vi "Main.vi"() -> ()   [LabVIEW 2022 SP3]
uses:
  States/FSM States V2.ctl
  <vilib>/express/express arith-compare/Formula/XNode/ExpressFormulaBlockNode.xnode
panel:
  out "Flag data log":i32=1 min=1 max=10 step=1
  out "Pitch positions (deg)":T1(graph)
  out "Yaw positions (deg)":T2(graph)
  in  "Start":bool
  in  "Load Button":bool
  in  "Default Button":bool
  out "Current state":T3
  in  "Stop button":bool
  in  "Tab Control":T4(tab)
  in  "Init Controller Parameters":T5={"Resolution level, N"=1, "Samples, re"=1, "Yaw gains"=[], "Pitch rate, mK"=[], "Yaw rate, mK"=[], "Pitch gains"=[], "Type controller, TC"=enum."PID"} {"Pitch gains" format="%.3f"; "Yaw rate, mK" format="%.2e"; "Pitch rate, mK" format="%.2e"; "Yaw gains" format="%.3f"; "Samples, re" min=1 max=100 step=1; "Resolution level, N" min=1 max=10 step=1}
  in  "Init Model Parameters":cluster{"States":dbl[]} {"States" format="%.3f"}
  in  "Init Wavenet-IIR Parameters":T6={"Activation function, fn"=0, "Neurons, J"=1, "Feedbacks, Q"=1, "Feedforwards, R"=1, "Inputs, I"=1, "Outputs, P"=1, "Weights, hW"=0.0, "Feedbacks, ha"=0.0, "Forwards, hb"=0.0, "Scalings, hA"=0.0, "Shiftings, hB"=0.0, "Persistan signal, ps"=0.0} {"Persistan signal, ps" format="%.2e"; "Shiftings, hB" format="%.2e"; "Scalings, hA" format="%.2e"; "Forwards, hb" format="%.2e"; "Feedbacks, ha" format="%.2e"; "Weights, hW" format="%.2e"; "Outputs, P" min=1 max=10 step=1; "Inputs, I" min=1 max=10 step=1; "Feedforwards, R" min=1 max=10 step=1; "Feedbacks, Q" min=1 max=10 step=1; "Neurons, J" min=1 max=99 step=1; "Activation function, fn" items=["Morlet", "RASP1", "RASP2", "RASP3", "POLYWOG1", "POLYWOG2", "POLYWOG3", "POLYWOG4", "POLYWOG5", "Shannon", "Atomic", "Flat top 1", "Flat top 2", "Flat top 3", "Flat top 4", "Flat top 5", "Flat top 6", "Hanning", "Hamming", "Blackman", "Blackman-Harris"]}
  out "Comparision, Errors":T7 {"costfnc" format="%_2f"; "Derry" format="%_2f"; "Derrp" format="%_2f"; "Dpy" format="%_2f"; "Dpe" format="%_2f"; "Cost func" scale=1.0..1000.0; "Yaw, err" scale=-3.0..3.0; "Pitch, err" scale=-3.0..3.0; "Yaw, e" scale=-3.0..3.0; "Pitch, e" scale=-3.0..3.0}
  out "Operation Parameters":T8={"Control signal, Vq"=0.0, "Control signal, Vf"=0.0, "Total control, U"=1.0, "Iteration, k"=1, "Period, T"=1.0, "Instant, kT"=1.0, "control Vpp"=0.0, "control Vpy"=0.0} {"control Vpy" format="%_2f"; "control Vpp" format="%_2f"; "Instant, kT" min=1.0 max=10.0 step=1.0 format="%.3f"; "Period, T" min=1.0 max=10.0 step=1.0 format="%.3f"; "Iteration, k" min=1 max=10 step=1; "Total control, U" min=1.0 max=10.0 step=1.0 format="%.3f"; "Control signal, Vf" scale=-30.0..30.0; "Control signal, Vq" scale=-30.0..30.0}
  in  "Desired Positions, yd":cluster{"Pitch, q":dbl, "Yaw, f":dbl}={"Pitch, q"=1.0, "Yaw, f"=1.0} {"Yaw, f" min=-40.0 max=40.0 step=5.0 format="%.2f"; "Pitch, q" min=-40.0 max=40.0 step=5.0 format="%.2f"}
  out "Acquisition, y":cluster{"Pitch, q":dbl, "Yaw, f":dbl}={"Pitch, q"=1.0, "Yaw, f"=1.0} {"Yaw, f" min=-40.0 max=40.0 step=5.0 format="%.2f"; "Pitch, q" min=-40.0 max=40.0 step=5.0 format="%.2f"}
  out "Approximation, ya":cluster{"Pitch, q":dbl, "Yaw, f":dbl}={"Pitch, q"=1.0, "Yaw, f"=1.0} {"Yaw, f" min=-40.0 max=40.0 step=5.0 format="%.2f"; "Pitch, q" min=-40.0 max=40.0 step=5.0 format="%.2f"}
  out "Model Parameters":cluster{"States (rad)":dbl[]} {"States (rad)" format="%.3f"}
  out "Controller Parameters":T5={"Resolution level, N"=1, "Samples, re"=1, "Yaw gains"=[], "Pitch rate, mK"=[], "Yaw rate, mK"=[], "Pitch gains"=[], "Type controller, TC"=enum."PID"} {"Pitch gains" format="%.3f"; "Yaw rate, mK" format="%.2e"; "Pitch rate, mK" format="%.2e"; "Yaw gains" format="%.3f"; "Samples, re" min=1 max=100 step=1; "Resolution level, N" min=1 max=10 step=1}
  in  "Wavenet-IIR Outputs":T9 {"Rho, R" format="%.3f"; "Gamma, G" format="%.3f"; "Estimated, y" format="%.3f"; "Neural, z" format="%.3f"}
  out "Wavenet-IIR Values":T10 {"Function, dy" format="%.3f"; "Function, y" format="%.3f"; "Tau, t" format="%.3f"; "Forwards, D" format="%.3f"; "Feedbacks, C" format="%.3f"; "Weights, W" format="%.3f"; "Shifts, B" format="%.3f"; "Scales, A" format="%.3f"}
  out "Wavenet-IIR Gradients":T11 {"Forwards, D" format="%.3f"; "Feedbacks, C" format="%.3f"; "Weights, W" format="%.3f"; "Shifts, B" format="%.3f"; "Scales, A" format="%.3f"}
  out "Wavenet-IIR Memories":T12 {"Activation functions, dF" format="%.3f"; "Wavenet, Z" format="%.3f"; "Tracking errors, e" format="%.3f"; "Activation functions, F" format="%.3f"; "Wavenet-IIR, Y" format="%.3f"}
  # "These values were propused by the designer."
  # "Value in radians and degrees."
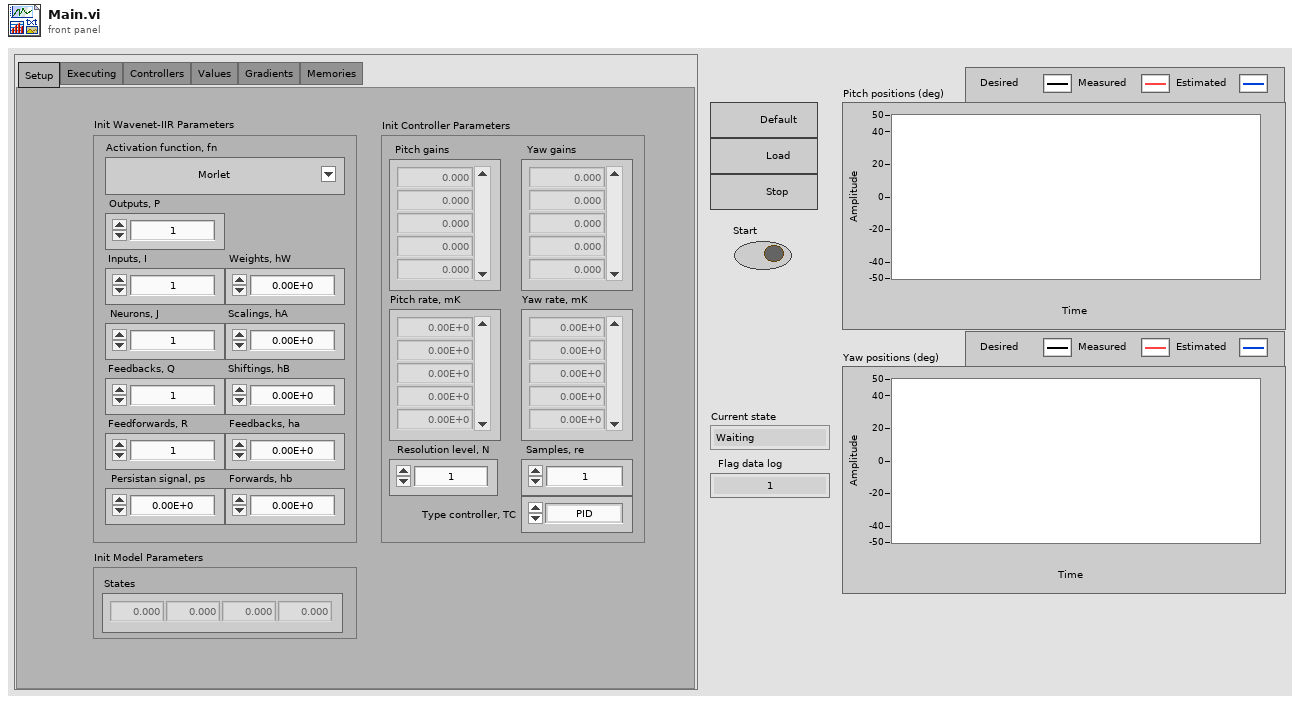
[diagram p1: front panel]
types:
  T1 = cluster{"Pitch, q":dbl, "Pitch, q":dbl, "Pitch, q":dbl}
  T2 = cluster{"Yaw, f":dbl, "Yaw, f":dbl, "Yaw, f":dbl}
  T3 = typedef "FSM States V2.ctl" = enum16{"Waiting", "Default configuration", "New configuration", "Boot parameters", "Execute", "Acquisition", "Wavelets", "WaveNet", "Filtering", "Comparision", "Gradients", "Datalog", "Update parameters", "Renew PID gains", "Renew PMR gains", "New PID signal", "New PMR signal", "Instant", "Time check", "Finish"}
  T4 = enum32{"Setup", "Executing", "Controllers", "Values", "Gradients", "Memories"}
  T5 = cluster{"Resolution level, N":i32, "Samples, re":i32, "Yaw gains":dbl[], "Pitch rate, mK":dbl[], "Yaw rate, mK":dbl[], "Pitch gains":dbl[], "Type controller, TC":enum16{"PID", "PMR"}}
  T6 = cluster{"Activation function, fn":u16, "Neurons, J":i32, "Feedbacks, Q":i32, "Feedforwards, R":i32, "Inputs, I":i32, "Outputs, P":i32, "Weights, hW":dbl, "Feedbacks, ha":dbl, "Forwards, hb":dbl, "Scalings, hA":dbl, "Shiftings, hB":dbl, "Persistan signal, ps":dbl}
  T7 = cluster{"Pitch, e":dbl, "Yaw, e":dbl, "Pitch, err":dbl, "Yaw, err":dbl, "Cost func":dbl, "Dpe":dbl, "Dpy":dbl, "Derrp":dbl, "Derry":dbl, "costfnc":dbl}
  T8 = cluster{"Control signal, Vq":dbl, "Control signal, Vf":dbl, "Total control, U":dbl, "Iteration, k":i32, "Period, T":dbl, "Instant, kT":dbl, "control Vpp":dbl, "control Vpy":dbl}
  T9 = cluster{"Neural, z":dbl[], "Estimated, y":dbl[], "Gamma, G":dbl[], "Rho, R":dbl[]}
  T10 = cluster{"Scales, A":dbl[], "Shifts, B":dbl[], "Weights, W":dbl[][], "Feedbacks, C":dbl[][], "Forwards, D":dbl[][], "Tau, t":dbl[], "Function, y":dbl[], "Function, dy":dbl[]}
  T11 = cluster{"Scales, A":dbl[], "Shifts, B":dbl[], "Weights, W":dbl[][], "Feedbacks, C":dbl[][], "Forwards, D":dbl[][]}
  T12 = cluster{"Wavenet-IIR, Y":dbl[][], "Activation functions, F":dbl[][], "Tracking errors, e":dbl[][], "Wavenet, Z":dbl[][], "Activation functions, dF":dbl[][]}
  T13 = cluster{"Pitch, q":dbl, "Pitch, q":dbl, "Numeric":dbl}[]
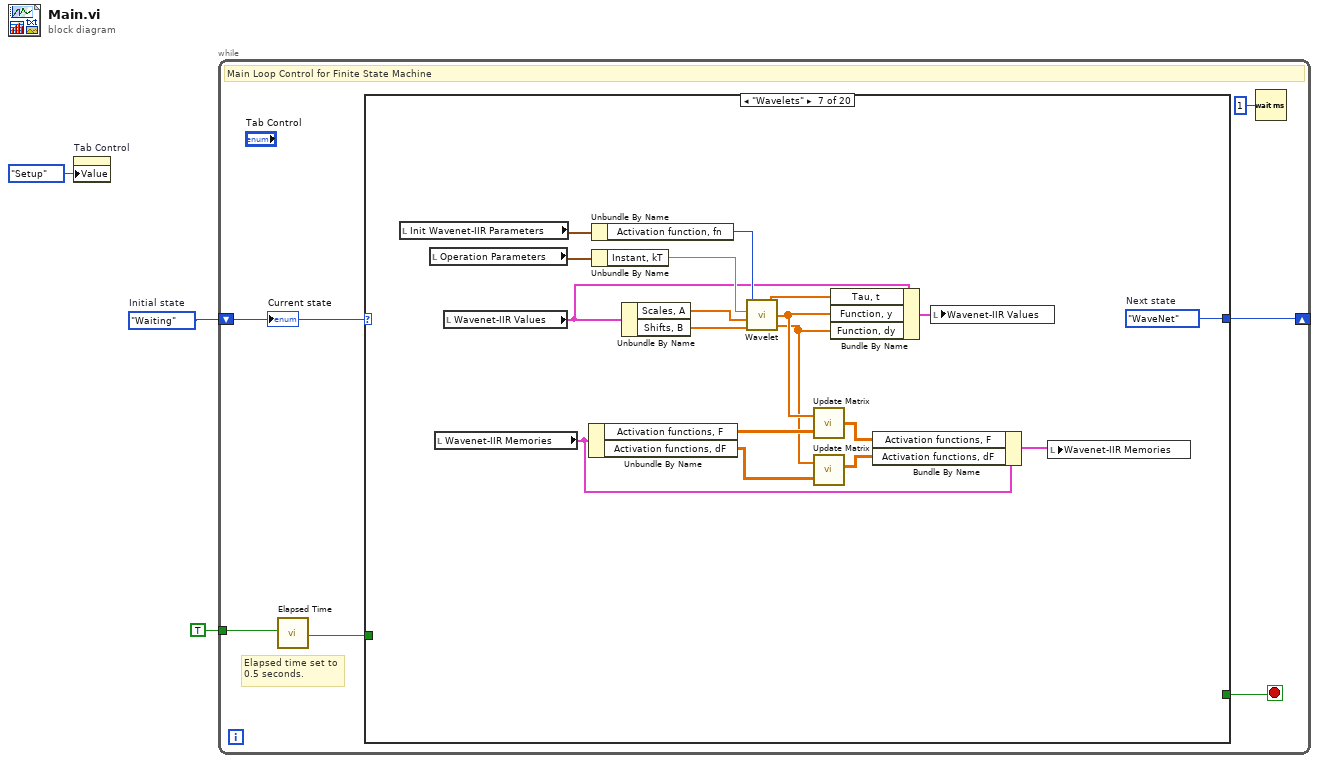
[diagram p0: block diagram]
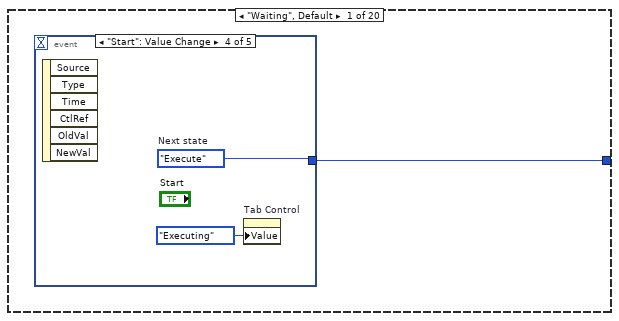
[diagram p2: hidden frame]
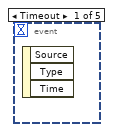
[diagram p3: hidden frame]
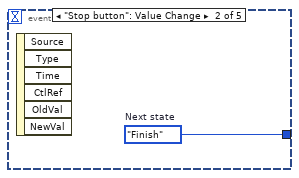
[diagram p4: hidden frame]
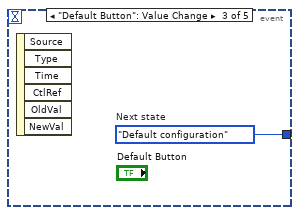
[diagram p5: hidden frame]
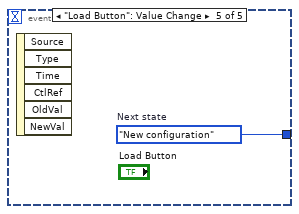
[diagram p6: hidden frame]
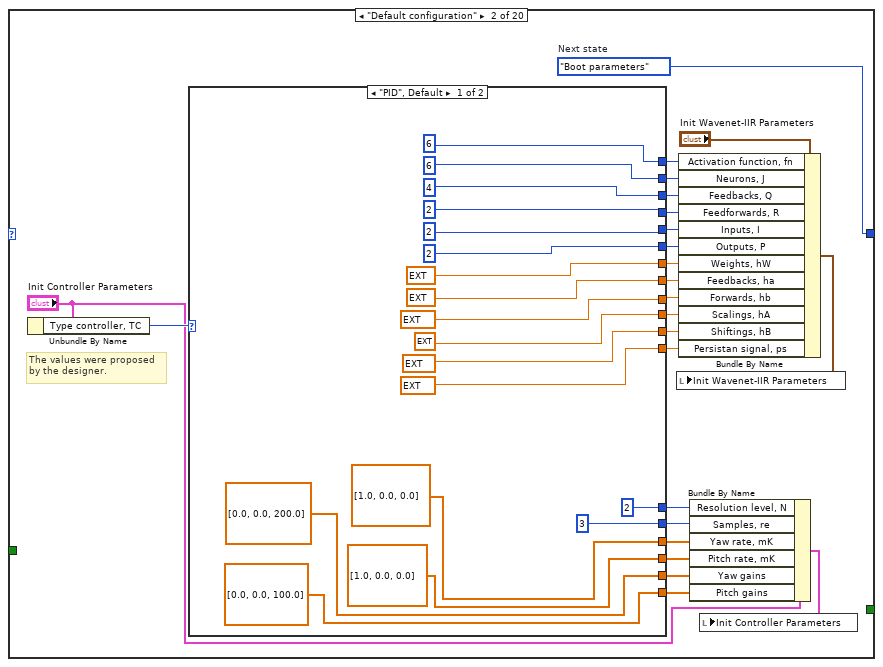
[diagram p7: hidden frame]
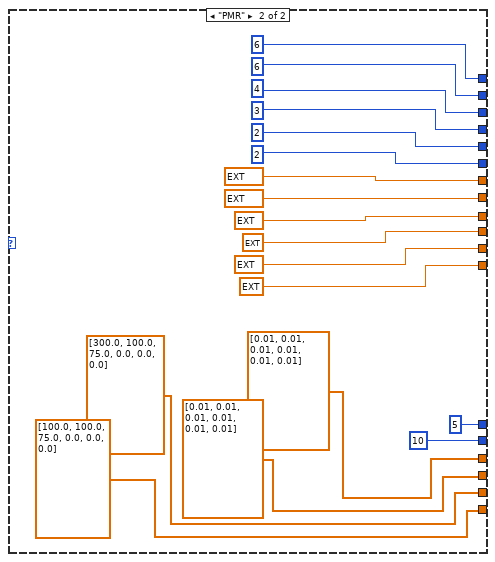
[diagram p8: hidden frame]
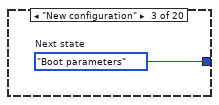
[diagram p9: hidden frame]
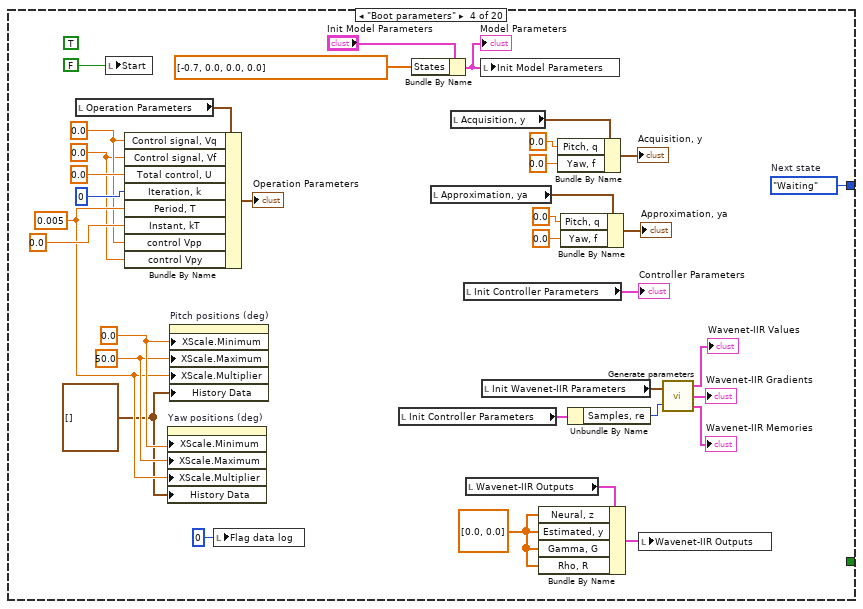
[diagram p10: hidden frame]
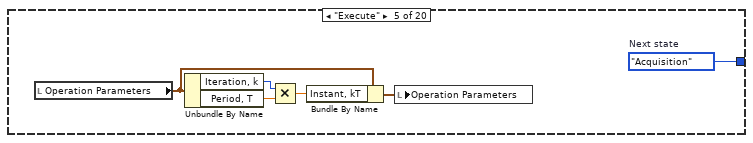
[diagram p11: hidden frame]
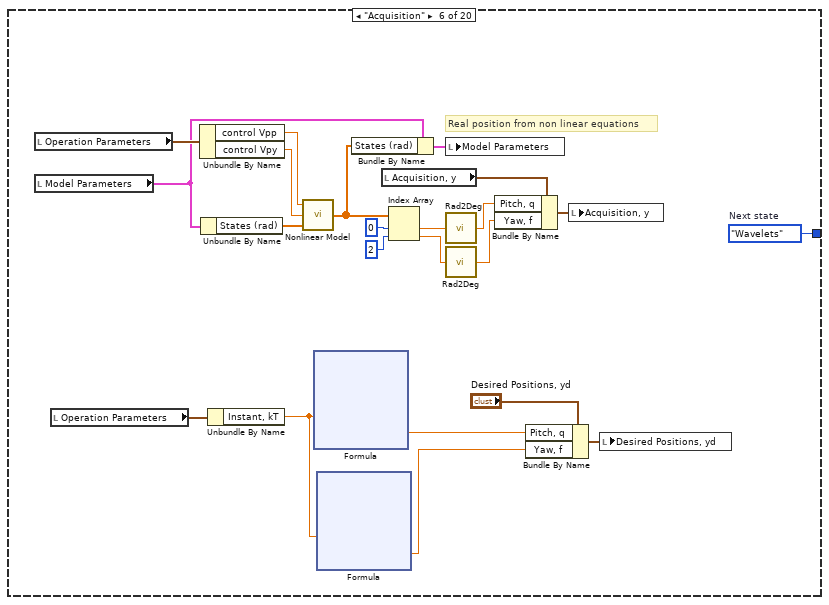
[diagram p12: hidden frame]
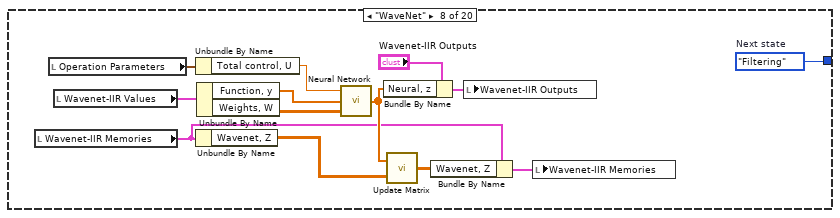
[diagram p13: hidden frame]
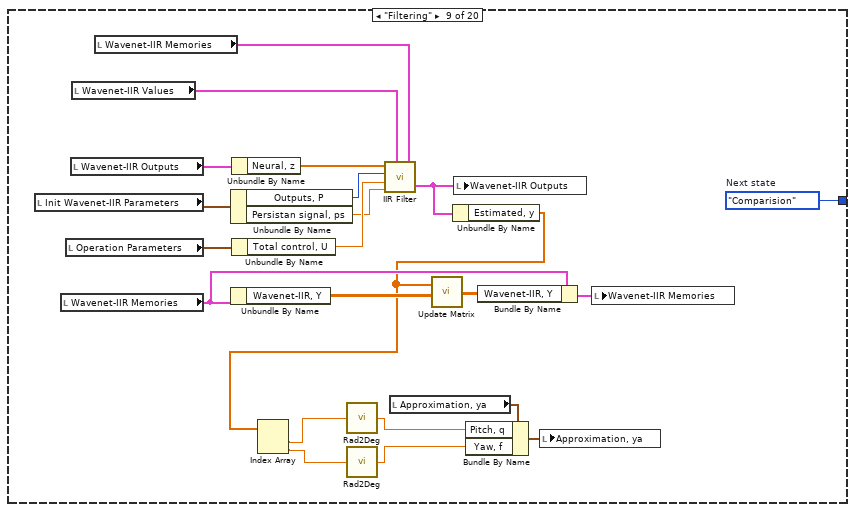
[diagram p14: hidden frame]
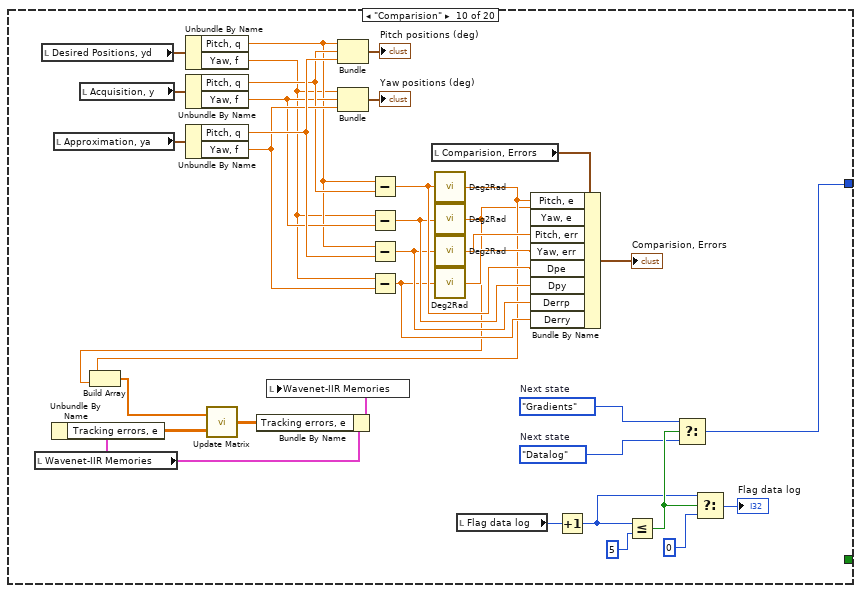
[diagram p15: hidden frame]
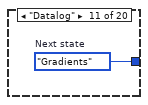
[diagram p16: hidden frame]
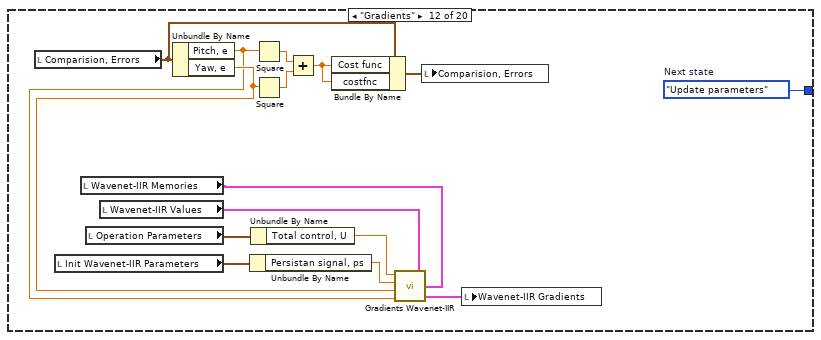
[diagram p17: hidden frame]
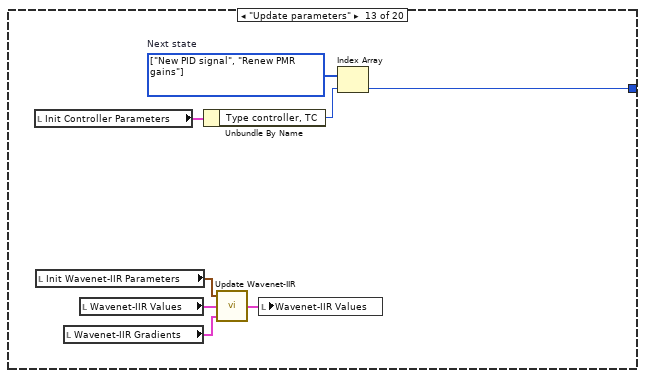
[diagram p18: hidden frame]
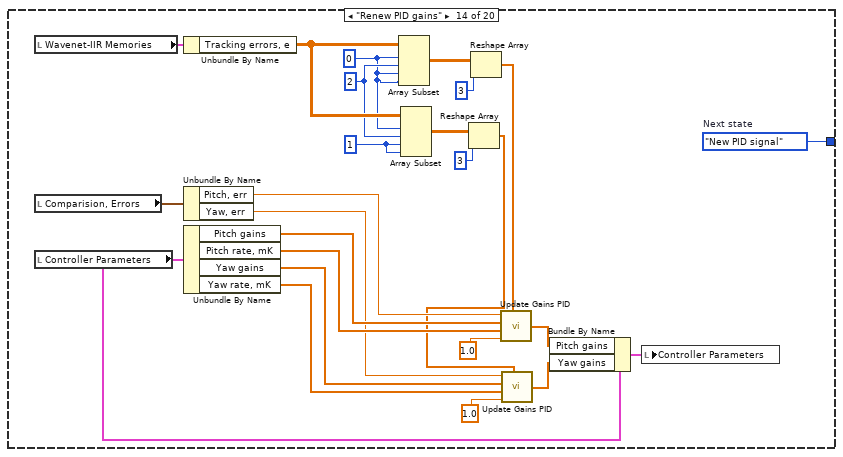
[diagram p19: hidden frame]
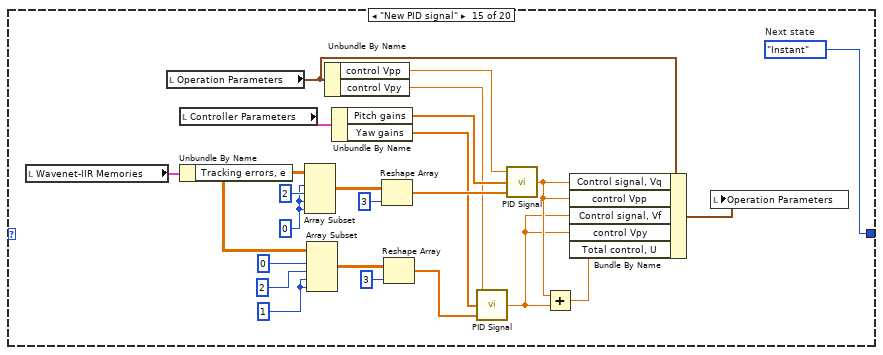
[diagram p20: hidden frame]
diagram:
  w3 = FSM_States_V2."Waiting"  # Initial state
  n1 = property on="Tab Control" class="TabCtl (strict)"("Value"=T4."Setup" ("Tab Control")) -> ()  [unwired: 2 in, 2 out]
  n2 = while {
    shift-right: [w6] -> _
    shift-left: w3 -> [w9]
    tunnel: TRUE ("Reset") -> [w8]
    stop <- w4 stop-if-true
    # "Elapsed time set to\n0.5 seconds."
    # "Main Loop Control for Finite State Machine"
    n3 = call "Elapsed Time"("Reset"=w8) -> ("Time has Elapsed"=w5:bool)  [unwired: 11 in, 7 out]
    n4 = case shown="\"Wavelets\"" w9 {
      tunnel: w5 -> [_ _ _ _ _ _ _ _ _ _ _ _ _ _ _ _ _ _ w325 _]
      tunnel: [w10 w28 w76 w111 w117 w139 w173 w186 w208 w221 w244 w259 w264 w292 w316 w317 w318 w319 w328 w329] -> w6
      tunnel: [_ _ _ _ _ _ _ _ _ _ _ _ _ _ _ _ _ _ "Stop button" TRUE ("Stop")] -> w4
      frame "Waiting", Default {
        n5 = event shown="[3] \"Start\": Value Change" {
          selector: _ -> [_ _ _ _ _]
          dyn-events: _ -> [_ _ _ _ _]
          timeout: _ -> [_ _ _ _ _]
          tunnel: [_ w11 w12 w14 w15] -> w10
          event Timeout {
            n6 = event-data() -> ()  [unwired: 1 in, 3 out]
          }
          event "Stop button": Value Change {
            w11 = FSM_States_V2."Finish"  # Next state
            n7 = event-data() -> ()  [unwired: 1 in, 6 out]
          }
          event "Default Button": Value Change {
            w12 = FSM_States_V2."Default configuration"  # Next state
            n8 = event-data() -> ()  [unwired: 1 in, 6 out]
          }
          event "Start": Value Change {
            w14 = FSM_States_V2."Execute"  # Next state
            n9 = event-data() -> ()  [unwired: 1 in, 6 out]
            n10 = property on="Tab Control" class="TabCtl (strict)"("Value"=T4."Executing" ("Tab Control")) -> ()  [unwired: 2 in, 2 out]
          }
          event "Load Button": Value Change {
            w15 = FSM_States_V2."New configuration"  # Next state
            n11 = event-data() -> ()  [unwired: 1 in, 6 out]
          }
        }
      }
      frame "Default configuration" {
        w28 = FSM_States_V2."Boot parameters"  # Next state
        # "The values were proposed\nby the designer."
        n12 = Unbundle By Name("Init Controller Parameters") -> ("Type controller, TC"=w39:enum16{"PID", "PMR"})
        n13 = case shown="\"PID\", Default" w39 {
          tunnel: [2 ("Resolution level, N") 5 ("Resolution level, N")] -> w37
          tunnel: [3 ("Forwards, R") 10 ("Forwards, R")] -> w35
          tunnel: [dbl[] [0.0, 0.0, 100.0] ("Yaw gains") dbl[] [100.0, 100.0, 75.0, 0.0, 0.0, 0.0] ("Yaw gains")] -> w34
          tunnel: [dbl[] [0.0, 0.0, 200.0] ("Yaw gains") dbl[] [300.0, 100.0, 75.0, 0.0, 0.0, 0.0] ("Yaw gains")] -> w33
          tunnel: [dbl[] [1.0, 0.0, 0.0] ("Yaw gains") dbl[] [0.01, 0.01, 0.01, 0.01, 0.01, 0.01] ("Yaw gains")] -> w32
          tunnel: [dbl[] [1.0, 0.0, 0.0] ("Yaw gains") dbl[] [0.01, 0.01, 0.01, 0.01, 0.01, 0.01] ("Yaw gains")] -> w31
          tunnel: [u16 6 ("Activation function, fn") u16 6 ("Activation function, fn")] -> w29
          tunnel: [6 ("Inputs, I") 6 ("Inputs, I")] -> w26
          tunnel: [4 ("Outputs, P") 4 ("Outputs, P")] -> w25
          tunnel: [2 ("Neurons, J") 3 ("Neurons, J")] -> w24
          tunnel: [2 ("Feedbacks, Q") 2 ("Feedbacks, Q")] -> w23
          tunnel: [2 ("Forwards, R") 2 ("Forwards, R")] -> w22
          tunnel: [ext 5.0000000000000000002e-7 ("Weights, hW") ext 0.0001 ("Weights, hW")] -> w21
          tunnel: [ext 0.00000100000000000000000004 ("Scaling, ha") ext 0.0001 ("Scaling, ha")] -> w20
          tunnel: [ext 1e-10 ("Shifting, hb") ext 5.0000000000000000002e-7 ("Shifting, hb")] -> w19
          tunnel: [ext 0.5 ("Feedbacks, ha") ext 0.5 ("Feedbacks, ha")] -> w18
          tunnel: [ext 0.005 ("Forwards, hb") ext 5.0000000000000000002e-7 ("Forwards, hb")] -> w17
          tunnel: [ext 1.00000000000000000003e-20 ("Persistent signal, sp") ext 100.0 ("Persistent signal, sp")] -> w16
          frame "PID", Default {
          }
          frame "PMR" {
          }
        }
        n14 = Bundle By Name(cluster="Init Wavenet-IIR Parameters", "Activation function, fn"=w29, "Neurons, J"=w26, "Feedbacks, Q"=w25, "Feedforwards, R"=w24, "Inputs, I"=w23, "Outputs, P"=w22, "Weights, hW"=w21, "Feedbacks, ha"=w20, "Forwards, hb"=w19, "Scalings, hA"=w18, "Shiftings, hB"=w17, "Persistan signal, ps"=w16) -> (w30:T6)
        n15 = local write "Init Wavenet-IIR Parameters"(w30) -> ()
        n16 = Bundle By Name(cluster="Init Controller Parameters", "Resolution level, N"=w37, "Samples, re"=w35, "Yaw rate, mK"=w31, "Pitch rate, mK"=w32, "Yaw gains"=w33, "Pitch gains"=w34) -> (w36:T5)
        n17 = local write "Init Controller Parameters"(w36) -> ()
      }
      frame "New configuration" {
        w76 = FSM_States_V2."Boot parameters"  # Next state
      }
      frame "Boot parameters" {
        w80 = T13 [] ("History Data")
        w82 = 50.0 ("X Scale.Range:Maximum")
        w83 = 0.0 ("X Scale.Range:Minimum")
        w84 = dbl[] [0.0, 0.0] ("Neural, z")
        w81 = 0.005 ("Period, T")
        w77 = 0.0 ("Control signal, Vf")
        w78 = 0.0 ("Control signal, Vq")
        w111 = FSM_States_V2."Waiting"  # Next state
        (unwired) TRUE ("Start LED")
        n18 = local read "Operation Parameters"() -> (w107:T8)
        n19 = local write "Start"(FALSE ("Start switch")) -> ()
        n20 = Bundle By Name(cluster=w107, "Control signal, Vq"=w78, "Control signal, Vf"=w77, "Total control, U"=0.0, "Iteration, k"=0, "Period, T"=w81, "Instant, kT"=0.0, "control Vpp"=w78, "control Vpy"=w77) -> (→"Operation Parameters":T8)
        n21 = property on="Yaw positions (deg)" class="WFChart (strict)"("XScale.Minimum"=w83, "XScale.Maximum"=w82, "XScale.Multiplier"=w81, "History Data"=w80) -> ()  [unwired: 2 in, 2 out]
        n22 = property on="Pitch positions (deg)" class="WFChart (strict)"("XScale.Minimum"=w83, "XScale.Maximum"=w82, "XScale.Multiplier"=w81, "History Data"=w80) -> ()  [unwired: 2 in, 2 out]
        n23 = local write "Flag data log"(0 ("Flag data log")) -> ()
        n24 = local read "Init Controller Parameters"() -> (w91:T5)
        n25 = Bundle By Name(cluster="Init Model Parameters", "States"=dbl[] [-0.7, 0.0, 0.0, 0.0]) -> (w94:cluster{"States":dbl[]})
        "Model Parameters" <- w94
        n26 = local read "Approximation, ya"() -> (w97:cluster{"Pitch, q":dbl, "Yaw, f":dbl})
        n27 = local read "Acquisition, y"() -> (w102:cluster{"Pitch, q":dbl, "Yaw, f":dbl})
        n28 = local read "Init Controller Parameters"() -> (→"Controller Parameters":T5)
        n29 = local read "Wavenet-IIR Outputs"() -> (w86:T9)
        n30 = local write "Init Model Parameters"(w94) -> ()
        n31 = local read "Init Wavenet-IIR Parameters"() -> (w92:T6)
        n32 = Bundle By Name(cluster=w86, "Neural, z"=w84, "Estimated, y"=w84, "Gamma, G"=w84, "Rho, R"=w84) -> (w85:T9)
        n33 = Bundle By Name(cluster=w102, "Pitch, q"=0.0, "Yaw, f"=0.0) -> (→"Acquisition, y":cluster{"Pitch, q":dbl, "Yaw, f":dbl})
        n34 = Bundle By Name(cluster=w97, "Pitch, q"=0.0, "Yaw, f"=0.0) -> (→"Approximation, ya":cluster{"Pitch, q":dbl, "Yaw, f":dbl})
        n35 = Unbundle By Name(w91) -> ("Samples, re"=w90:i32)
        n36 = local write "Wavenet-IIR Outputs"(w85) -> ()
        n37 = call "Generate parameters.vi"("Wavenet-IIR Parameters"=w92, "Samples, re"=w90) -> ("Wavenet-IIR Behavior"=→"Wavenet-IIR Values":T10, "Wavenet-IIR Gradients"=→"Wavenet-IIR Gradients":T11, "Wavenet-IIR Memories"=→"Wavenet-IIR Memories":T12)
      }
      frame "Execute" {
        w117 = FSM_States_V2."Acquisition"  # Next state
        n38 = local read "Operation Parameters"() -> (w114:T8)
        n39 = Unbundle By Name(w114) -> ("Iteration, k"=w116:i32, "Period, T"=w115:dbl)
        n40 = Multiply(x=w116, y=w115) -> (x*y=w113:dbl)
        n41 = Bundle By Name(cluster=w114, "Instant, kT"=w113) -> (w112:T8)
        n42 = local write "Operation Parameters"(w112) -> ()
      }
      frame "Acquisition" {
        w139 = FSM_States_V2."Wavelets"  # Next state
        # "Real position from non linear equations"
        n43 = local read "Operation Parameters"() -> (w138:T8)
        n44 = local read "Model Parameters"() -> (w134:cluster{"States (rad)":dbl[]})
        n45 = local read "Operation Parameters"() -> (w123:T8)
        n46 = Unbundle By Name(w138) -> ("control Vpp"=w137:dbl, "control Vpy"=w136:dbl)
        n47 = Unbundle By Name(w134) -> ("States (rad)"=w135:dbl[])
        n48 = Unbundle By Name(w123) -> ("Instant, kT"=w121:dbl)
        n49 = call "Nonlinear Model.vi"("State variables, x"=w135, "Contro yaw, f"=w136, "Control pitch, q"=w137) -> ("New state variables"=w124:dbl[])
        n50 = xnode "Formula"("kT"=w121) -> ("Result"=w119:dbl)  [unwired: 1 in, 1 out]
        n51 = xnode "Formula"("kT"=w121) -> ("Result"=w118:dbl)  [unwired: 1 in, 1 out]
        n52 = Bundle By Name(cluster=w134, "States (rad)"=w124) -> (w133:cluster{"States (rad)":dbl[]})
        n53 = local read "Acquisition, y"() -> (w131:cluster{"Pitch, q":dbl, "Yaw, f":dbl})
        n54 = Index Array(array=w124, index #1=0 ("index"), index #2=2 ("index")) -> (element #1=w126:dbl, element #2=w125:dbl)
        n55 = local write "Model Parameters"(w133) -> ()
        n56 = call "Rad2Deg.vi"("Input"=w126) -> ("Output"=w130:dbl)
        n57 = call "Rad2Deg.vi"("Input"=w125) -> ("Output"=w129:dbl)
        n58 = Bundle By Name(cluster=w131, "Pitch, q"=w130, "Yaw, f"=w129) -> (w132:cluster{"Pitch, q":dbl, "Yaw, f":dbl})
        n59 = Bundle By Name(cluster="Desired Positions, yd", "Pitch, q"=w119, "Yaw, f"=w118) -> (w122:cluster{"Pitch, q":dbl, "Yaw, f":dbl})
        n60 = local write "Acquisition, y"(w132) -> ()
        n61 = local write "Desired Positions, yd"(w122) -> ()
      }
      frame "Wavelets" {
        w173 = FSM_States_V2."WaveNet"  # Next state
        n62 = local read "Init Wavenet-IIR Parameters"() -> (w172:T6)
        n63 = local read "Operation Parameters"() -> (w170:T8)
        n64 = local read "Wavenet-IIR Memories"() -> (w158:T12)
        n65 = local read "Wavenet-IIR Values"() -> (w165:T10)
        n66 = Unbundle By Name(w158) -> ("Activation functions, F"=w163:dbl[][], "Activation functions, dF"=w162:dbl[][])
        n67 = Unbundle By Name(w172) -> ("Activation function, fn"=w171:u16)
        n68 = Unbundle By Name(w170) -> ("Instant, kT"=w169:dbl)
        n69 = Unbundle By Name(w165) -> ("Scales, A"=w168:dbl[], "Shifts, B"=w167:dbl[])
        n70 = call "Wavelet.vi"("Shifts, b"=w167, "Scales, a"=w168, "Instant, kT"=w169, "Activation function, fn"=w171) -> ("Function, dy"=w160:dbl[], "Function, y"=w161:dbl[], "Tau, t"=w166:dbl[])
        n71 = call "Update Matrix.vi"("Older"=w163, "Current"=w161) -> ("New"=w157:dbl[][])
        n72 = call "Update Matrix.vi"("Older"=w162, "Current"=w160) -> ("New"=w156:dbl[][])
        n73 = Bundle By Name(cluster=w165, "Tau, t"=w166, "Function, y"=w161, "Function, dy"=w160) -> (w164:T10)
        n74 = Bundle By Name(cluster=w158, "Activation functions, F"=w157, "Activation functions, dF"=w156) -> (w159:T12)
        n75 = local write "Wavenet-IIR Values"(w164) -> ()
        n76 = local write "Wavenet-IIR Memories"(w159) -> ()
      }
      frame "WaveNet" {
        w186 = FSM_States_V2."Filtering"  # Next state
        n77 = local read "Wavenet-IIR Memories"() -> (w179:T12)
        n78 = local read "Operation Parameters"() -> (w175:T8)
        n79 = local read "Wavenet-IIR Values"() -> (w184:T10)
        n80 = Unbundle By Name(w175) -> ("Total control, U"=w174:dbl)
        n81 = Unbundle By Name(w179) -> ("Wavenet, Z"=w181:dbl[][])
        n82 = Unbundle By Name(w184) -> ("Function, y"=w176:dbl[], "Weights, W"=w185:dbl[][])
        n83 = call "Neural Network.vi"("Weights, W"=w185, "Function, y"=w176, "Control, U"=w174) -> ("Outputs, z"=w182:dbl[])
        n84 = Bundle By Name(cluster="Wavenet-IIR Outputs", "Neural, z"=w182) -> (w183:T9)
        n85 = call "Update Matrix.vi"("Older"=w181, "Current"=w182) -> ("New"=w178:dbl[][])
        n86 = Bundle By Name(cluster=w179, "Wavenet, Z"=w178) -> (w180:T12)
        n87 = local write "Wavenet-IIR Outputs"(w183) -> ()
        n88 = local write "Wavenet-IIR Memories"(w180) -> ()
      }
      frame "Filtering" {
        w208 = FSM_States_V2."Comparision"  # Next state
        n89 = local read "Init Wavenet-IIR Parameters"() -> (w205:T6)
        n90 = local read "Wavenet-IIR Memories"() -> (w196:T12)
        n91 = local read "Operation Parameters"() -> (w203:T8)
        n92 = local read "Wavenet-IIR Outputs"() -> (w207:T9)
        n93 = local read "Wavenet-IIR Values"() -> (w200:T10)
        n94 = local read "Wavenet-IIR Memories"() -> (w199:T12)
        n95 = Unbundle By Name(w205) -> ("Outputs, P"=w204:i32, "Persistan signal, ps"=w201:dbl)
        n96 = Unbundle By Name(w196) -> ("Wavenet-IIR, Y"=w197:dbl[][])
        n97 = Unbundle By Name(w207) -> ("Neural, z"=w206:dbl[])
        n98 = Unbundle By Name(w203) -> ("Total control, U"=w202:dbl)
        n99 = call "IIR Filter.vi"("Neural, z"=w206, "Outputs, P"=w204, "Total control, U"=w202, "Persistant signal, ps"=w201, "Wavenet-IIR Values"=w200, "Wavenet-IIR Memories"=w199) -> ("Wavenet-IIR Outputs"=w198:T9)
        n100 = local read "Approximation, ya"() -> (w192:cluster{"Pitch, q":dbl, "Yaw, f":dbl})
        n101 = Unbundle By Name(w198) -> ("Estimated, y"=w187:dbl[])
        n102 = Index Array(array=w187) -> (element #1=w189:dbl, element #2=w188:dbl)  [unwired: 2 in]
        n103 = call "Rad2Deg.vi"("Input"=w189) -> ("Output"=w191:dbl)
        n104 = call "Rad2Deg.vi"("Input"=w188) -> ("Output"=w190:dbl)
        n105 = call "Update Matrix.vi"("Older"=w197, "Current"=w187) -> ("New"=w195:dbl[][])
        n106 = local write "Wavenet-IIR Outputs"(w198) -> ()
        n107 = Bundle By Name(cluster=w192, "Pitch, q"=w191, "Yaw, f"=w190) -> (w193:cluster{"Pitch, q":dbl, "Yaw, f":dbl})
        n108 = Bundle By Name(cluster=w196, "Wavenet-IIR, Y"=w195) -> (w194:T12)
        n109 = local write "Approximation, ya"(w193) -> ()
        n110 = local write "Wavenet-IIR Memories"(w194) -> ()
      }
      frame "Comparision" {
        w222 = FSM_States_V2."Datalog"  # Next state
        w223 = FSM_States_V2."Gradients"  # Next state
        n111 = local read "Wavenet-IIR Memories"() -> (w213:T12)
        n112 = local read "Desired Positions, yd"() -> (w243:cluster{"Pitch, q":dbl, "Yaw, f":dbl})
        n113 = Unbundle By Name(w213) -> ("Tracking errors, e"=w218:dbl[][])
        n114 = local read "Approximation, ya"() -> (w241:cluster{"Pitch, q":dbl, "Yaw, f":dbl})
        n115 = local read "Acquisition, y"() -> (w242:cluster{"Pitch, q":dbl, "Yaw, f":dbl})
        n116 = Unbundle By Name(w243) -> ("Pitch, q"=w210:dbl, "Yaw, f"=w209:dbl)
        n117 = Unbundle By Name(w242) -> ("Pitch, q"=w212:dbl, "Yaw, f"=w211:dbl)
        n118 = Unbundle By Name(w241) -> ("Pitch, q"=w231:dbl, "Yaw, f"=w230:dbl)
        n119 = Bundle("Pitch, q"=w210, "Pitch, q"=w212, "Pitch, q"=w231) -> (→"Pitch positions (deg)":T1)  [unwired: 1 in]
        n120 = Bundle("Yaw, f"=w209, "Yaw, f"=w211, "Yaw, f"=w230) -> (→"Yaw positions (deg)":T2)  [unwired: 1 in]
        n121 = Subtract(x=w210, y=w212) -> (x-y=w235:dbl)
        n122 = Subtract(x=w209, y=w211) -> (x-y=w234:dbl)
        n123 = Subtract(x=w210, y=w231) -> (x-y=w233:dbl)
        n124 = Subtract(x=w209, y=w230) -> (x-y=w232:dbl)
        n125 = local read "Comparision, Errors"() -> (w238:T7)
        n126 = call "Deg2Rad.vi"("Input"=w235) -> ("Output"=w216:dbl)
        n127 = call "Deg2Rad.vi"("Input"=w234) -> ("Output"=w215:dbl)
        n128 = Build Array(w216, w215) -> (w217:dbl[])
        n129 = call "Update Matrix.vi"("Older"=w218, "Current"=w217) -> ("New"=w214:dbl[][])
        n130 = Bundle By Name(cluster=w213, "Tracking errors, e"=w214) -> (w219:T12)
        n131 = local write "Wavenet-IIR Memories"(w219) -> ()
        n132 = call "Deg2Rad.vi"("Input"=w233) -> ("Output"=w237:dbl)
        n133 = call "Deg2Rad.vi"("Input"=w232) -> ("Output"=w236:dbl)
        n134 = local read "Flag data log"() -> (w224:i32)
        n135 = Bundle By Name(cluster=w238, "Pitch, e"=w216, "Yaw, e"=w215, "Pitch, err"=w237, "Yaw, err"=w236, "Dpe"=w235, "Dpy"=w234, "Derrp"=w233, "Derry"=w232) -> (→"Comparision, Errors":T7)
        n136 = Increment(x=w224) -> (x+1=w225:i32)
        n137 = Less Or Equal?(x=w225, y=5) -> (x <= y?=w226:bool)
        n138 = Select(t=w223, s=w226, f=w222) -> (s? t:f=w221:T3)
        n139 = Select(t=w225, s=w226, f=0) -> (s? t:f=→"Flag data log":i32)
      }
      frame "Datalog" {
        w244 = FSM_States_V2."Gradients"  # Next state
      }
      frame "Gradients" {
        w259 = FSM_States_V2."Update parameters"  # Next state
        n140 = local read "Comparision, Errors"() -> (w256:T7)
        n141 = local read "Init Wavenet-IIR Parameters"() -> (w249:T6)
        n142 = local read "Wavenet-IIR Memories"() -> (w246:T12)
        n143 = local read "Operation Parameters"() -> (w253:T8)
        n144 = local read "Wavenet-IIR Values"() -> (w247:T10)
        n145 = Unbundle By Name(w256) -> ("Pitch, e"=w250:dbl, "Yaw, e"=w251:dbl)
        n146 = Unbundle By Name(w249) -> ("Persistan signal, ps"=w248:dbl)
        n147 = Unbundle By Name(w253) -> ("Total control, U"=w252:dbl)
        n148 = Square(x=w250) -> (x^2=w258:dbl)
        n149 = Square(x=w251) -> (x^2=w257:dbl)
        n150 = Add(x=w258, y=w257) -> (x+y=w255:dbl)
        n151 = Bundle By Name(cluster=w256, "Cost func"=w255, "costfnc"=w255) -> (w254:T7)
        n152 = call "Gradients Wavenet-IIR.vi"("Wavenet-IIR Memories"=w246, "Wavenet-IIR Values"=w247, "Pitch, e"=w250, "Yaw, e"=w251, "Persistant signal"=w248, "Total control, U"=w252) -> ("Wavenet-IIR Gradients"=w245:T11)
        n153 = local write "Comparision, Errors"(w254) -> ()
        n154 = local write "Wavenet-IIR Gradients"(w245) -> ()
      }
      frame "Update parameters" {
        w267 = T3[] [enum."New PID signal", enum."Renew PMR gains"] items=["Waiting", "Default configuration", "New configuration", "Boot parameters", "Execute", "Acquisition", "Wavelets", "WaveNet", "Filtering", "Comparision", "Gradients", "Datalog", "Update parameters", "Renew PID gains", "Renew PMR gains", "New PID signal", "New PMR signal", "Instant", "Time check", "Finish"]  # Next state
        n155 = local read "Init Controller Parameters"() -> (w266:T5)
        n156 = local read "Init Wavenet-IIR Parameters"() -> (w261:T6)
        n157 = local read "Wavenet-IIR Gradients"() -> (w262:T11)
        n158 = local read "Wavenet-IIR Values"() -> (w263:T10)
        n159 = Unbundle By Name(w266) -> ("Type controller, TC"=w265:enum16{"PID", "PMR"})
        n160 = call "Update Wavenet-IIR.vi"("Wavenet-IIR Gradients"=w262, "Wavenet-IIR Older"=w263, "Wavenet-IIR Parameters"=w261) -> ("Wavenet-IIR New"=w260:T10)
        n161 = local write "Wavenet-IIR Values"(w260) -> ()
        n162 = Index Array(array=w267, index=w265) -> (element=w264:T3)
      }
      frame "Renew PID gains" {
        w274 = 1 ("column 1")
        w276 = 2 ("row N")
        w275 = 0 ("row 1")
        w292 = FSM_States_V2."New PID signal"  # Next state
        n163 = local read "Wavenet-IIR Memories"() -> (w278:T12)
        n164 = local read "Comparision, Errors"() -> (w288:T7)
        n165 = local read "Controller Parameters"() -> (w286:T5)
        n166 = Unbundle By Name(w278) -> ("Tracking errors, e"=w277:dbl[][])
        n167 = Unbundle By Name(w288) -> ("Pitch, err"=w287:dbl, "Yaw, err"=w283:dbl)
        n168 = Unbundle By Name(w286) -> ("Pitch gains"=w291:dbl[], "Pitch rate, mK"=w290:dbl[], "Yaw gains"=w282:dbl[], "Yaw rate, mK"=w281:dbl[])
        n169 = Array Subset(array=w277, index (row)=w275, length (row)=w276, index (col)=w275, length (col)=w275) -> (w273:dbl[][])
        n170 = Array Subset(array=w277, index (row)=w275, length (row)=w276, index (col)=w274, length (col)=w274) -> (w270:dbl[][])
        n171 = Reshape Array(w270, 3 ("dimension size")) -> (w268:dbl[])
        n172 = Reshape Array(w273, 3 ("dimension size")) -> (w269:dbl[])
        n173 = call "Update Gains PID.vi"("Error, e"=w287, "Gains, Kp"=w291, "Update rate, mK"=w290, "Gamma, G"=1.0, "Tracking errors, e"=w269) -> ("New gains, Kp"=w284:dbl[])
        n174 = call "Update Gains PID.vi"("Error, e"=w283, "Gains, Kp"=w282, "Update rate, mK"=w281, "Gamma, G"=1.0, "Tracking errors, e"=w268) -> ("New gains, Kp"=w279:dbl[])
        n175 = Bundle By Name(cluster=w286, "Pitch gains"=w284, "Yaw gains"=w279) -> (w285:T5)
        n176 = local write "Controller Parameters"(w285) -> ()
      }
      frame "New PID signal" {
        w299 = 1 ("row N")
        w310 = 0 ("row 1")
        w316 = FSM_States_V2."Instant"  # Next state
        n177 = local read "Wavenet-IIR Memories"() -> (w312:T12)
        n178 = local read "Operation Parameters"() -> (w306:T8)
        n179 = local read "Controller Parameters"() -> (w315:T5)
        n180 = Unbundle By Name(w312) -> ("Tracking errors, e"=w302:dbl[][])
        n181 = Array Subset(array=w302, index (row)=w310, length (row)=2 ("row N"), index (col)=w310, length (col)=w310) -> (w309:dbl[][])
        n182 = Array Subset(array=w302, index (row)=0 ("row 1"), length (row)=2 ("row N"), index (col)=w299, length (col)=w299) -> (w303:dbl[][])
        n183 = Unbundle By Name(w306) -> ("control Vpp"=w313:dbl, "control Vpy"=w296:dbl)
        n184 = Unbundle By Name(w315) -> ("Pitch gains"=w314:dbl[], "Yaw gains"=w297:dbl[])
        n185 = Reshape Array(w309, 3 ("dimension size")) -> (w307:dbl[])
        n186 = Reshape Array(w303, 3 ("dimension size")) -> (w298:dbl[])
        n187 = call "PID Signal.vi"("Tracking errors, e"=w298, "Gains, Ks"=w297, "Control, u(k)"=w296) -> ("Control, u(k+1)"=w293:dbl)
        n188 = call "PID Signal.vi"("Tracking errors, e"=w307, "Gains, Ks"=w314, "Control, u(k)"=w313) -> ("Control, u(k+1)"=w294:dbl)
        n189 = Add(x=w294, y=w293) -> (x+y=w295:dbl)
        n190 = Bundle By Name(cluster=w306, "Control signal, Vq"=w294, "control Vpp"=w294, "Control signal, Vf"=w293, "control Vpy"=w293, "Total control, U"=w295) -> (w305:T8)
        n191 = local write "Operation Parameters"(w305) -> ()
      }
      frame "Renew PMR gains" {
        w317 = FSM_States_V2."New PMR signal"  # Next state
      }
      frame "New PMR signal" {
        w318 = FSM_States_V2."Instant"  # Next state
      }
      frame "Instant" {
        w319 = FSM_States_V2."Execute"  # Next state
        n192 = local read "Operation Parameters"() -> (w320:T8)
        n193 = Unbundle By Name(w320) -> ("Iteration, k"=w322:i32)
        n194 = Increment(x=w322) -> (x+1=w321:i32)
        n195 = Bundle By Name(cluster=w320, "Iteration, k"=w321) -> (w323:T8)
        n196 = local write "Operation Parameters"(w323) -> ()
      }
      frame "Time check" {
        w326 = FSM_States_V2."Time check"  # Next state
        w327 = FSM_States_V2."Instant"  # Next state
        n197 = Select(t=w327, s=w325, f=w326) -> (s? t:f=w328:T3)
      }
      frame "Finish" {
        w329 = FSM_States_V2."Finish"  # Next state
      }
    }
    n198 = Wait (ms)(milliseconds to wait=u32 1) -> ()  [unwired: 1 out]
    "Current state" <- w9
  }
